vi "Write Input Registers.vi"(8 "error in (no error)":errorcluster, 9 "register values":u16[](array[numeric]), 10 "starting address":u16, 11 "Standard Data Model in":refnum<class "Standard Data Model.lvclass">) -> (0 "error out":errorcluster, 3 "Standard Data Model out":refnum<class "Standard Data Model.lvclass">)   [LabVIEW 2013, in "Modbus Library - Advance.lvlib" / "Standard Data Model.lvclass"]
doc: "Writes the values of multiple input register values in series, starting at address M."
uses:
  Standard Data Model.lvclass
  Standard Data Model.lvclass/Standard Data Model.ctl
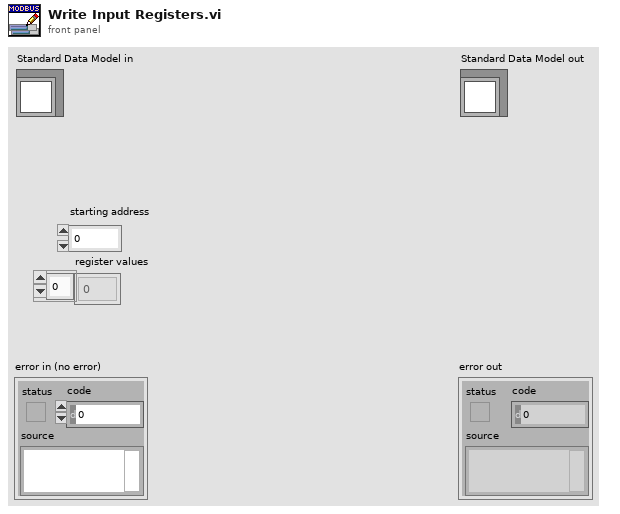
[diagram p1: front panel]
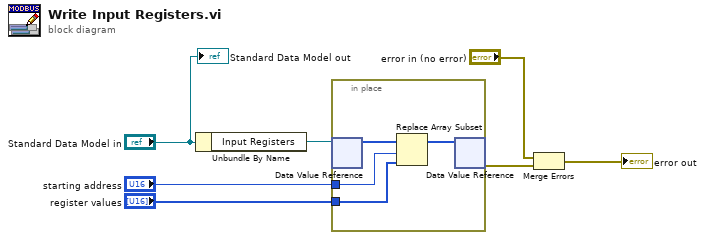
[diagram p0: block diagram]
diagram:
  n1 = Unbundle By Name("Standard Data Model in") -> ("Input Registers"=w4:refnum<data-value>)
  n2 = in-place {
    in-place-border: "starting address" -> [w11]
    in-place-border: "register values" -> [w10]
    n3 = in-place-dvr #1(w4) -> (w9:u16[])  [unwired: 1 out]
    n4 = Replace Array Subset(array=w9, new element=w10, index=w11) -> (w8:u16[])
    n5 = in-place-dvr #1(w8) -> (w1:errorcluster)  [unwired: 1 out]
  }
  n6 = Merge Errors("error in (no error)", w1) -> (→"error out":errorcluster)
  "Standard Data Model out" <- "Standard Data Model in"
